vi "Pre Launch Init.vi"(11 "RootModel in":refnum<class "RootModel.lvclass">) -> (0 "error out":errorcluster, 3 "RootModel out":refnum<class "RootModel.lvclass">)   [LabVIEW 2020, in "RootModel.lvlib" / "RootModel.lvclass"]
doc: "(<B>Filename</B>: Actor Framework.lvlib:Actor.lvclass:Pre Launch Init.vi)\n\nDefines behavior that occurs after the Launch Nested Actor method is invoked but before the actor's Actor Core method begins running.\n\nBy default, this method does nothing. A descendant class may override it to define behavior."
uses:
  RootModel.lvclass
  C:/Program Files/National Instruments/LabVIEW 2020/vi.lib/ActorFramework/Actor/Actor.lvclass
  RootModel.lvclass/RootModel.ctl
  <vilib>/ActorFramework/Actor/Actor.lvclass/Actor.ctl
  <vilib>/ActorFramework/Message Enqueuer/Message Enqueuer.lvclass/Message Enqueuer.ctl
  <vilib>/ActorFramework/Message Enqueuer/Message Priority.ctl
  <vilib>/ActorFramework/Message Enqueuer/Init from Existing Queue.vi
  <vilib>/ActorFramework/Message Priority Queue/Priority Enqueue.vi
  <vilib>/ActorFramework/Message Enqueuer/Message Enqueuer.lvclass
  IModel/IModel/IModel.lvclass
  RootModel Messages/Run Headless Msg/Run Headless Msg.lvclass
  <vilib>/ActorFramework/Actor/Actor.lvclass
  C:/Program Files/National Instruments/LabVIEW 2020/vi.lib/ActorFramework/Message/Message.lvclass
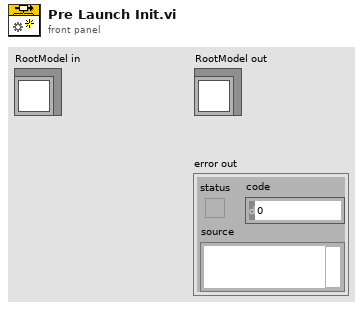
[diagram p1: front panel]
types:
  T1 = typedef "Actor Framework.lvlib/Message Enqueuer.lvclass/Message Priority.ctl" = enum16{"Low", "Normal", "High"}
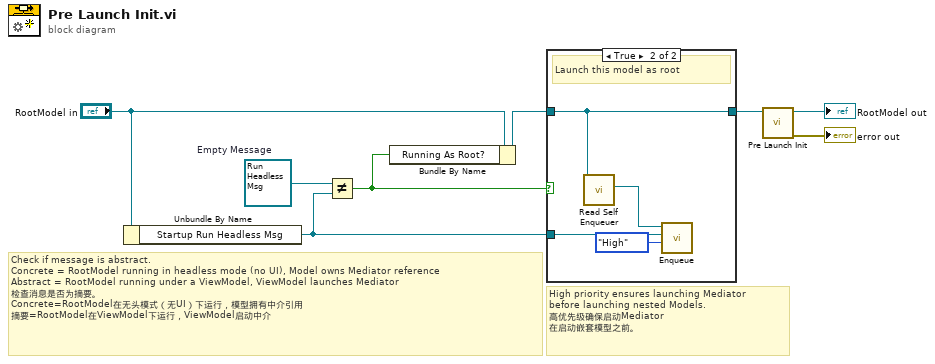
[diagram p0: block diagram]
diagram:
  w7 = refnum<class "Run Headless Msg.lvclass"> refnum  # Empty Message
  # "High priority ensures launching Mediator\nbefore launching nested Models.\n高优先级确保启动Mediator\n在启动嵌套模型之前。"
  # "Check if message is abstract.\nConcrete = RootModel running in headless mode (no UI), Model owns Mediator reference\nAbstract = RootModel running under a ViewModel, ViewModel launches Mediator\n检查消息是否为摘要。\nConcrete=RootModel在无头模式（无UI）下运行，模型拥有中介引用\n摘要=RootModel在ViewModel下运行，ViewModel启动中介"
  n1 = Unbundle By Name("RootModel in") -> ("Startup Run Headless Msg"=w5:refnum<class "Run Headless Msg.lvclass">)
  n2 = Not Equal?(x=w7, y=w5) -> (x != y?=w1:bool)
  n3 = Bundle By Name(cluster="RootModel in", "Running As Root?"=w1) -> (w2:refnum<class "RootModel.lvclass">)
  n4 = case shown="True" w1 {
    tunnel: w5 -> [_ w13]
    tunnel: w2 -> [w9 w10]
    tunnel: [w9 w10] -> w3
    frame False {
      # "NOT running as root"
    }
    frame True {
      # "Launch this model as root"
      n5 = call <vilib>:"Read Self Enqueuer.vi"("Actor"=w10) -> ("Self Enqueuer"=w11:refnum<class "Message Enqueuer.lvclass">)  [unwired: 10 in]
      n6 = call <vilib>:"Enqueue.vi"("Message Priority (Normal)"=Message_Priority."High", "Message"=w13, "Message Enqueuer in"=w11) -> ()  [unwired: 7 in, 2 out]
    }
  }
  n7 = call-parent "Pre Launch Init.vi"("IModel in"=w3) -> ("error out"=→"error out":errorcluster, "IModel out"=→"RootModel out":refnum<class "RootModel.lvclass">)  [unwired: 9 in]
